vi "Open Hardware.vi"(8 "error in (no error)":errorcluster, 11 "Instrument.Oxford1820 in":refnum<class "Instrument.Oxford1820.lvclass">) -> (0 "error out":errorcluster, 3 "Instrument.Oxford1820 out":refnum<class "Instrument.Oxford1820.lvclass">)   [LabVIEW 2019, in "Instrument.Oxford1820.lvclass"]
uses:
  Instrument.Oxford1820.lvclass
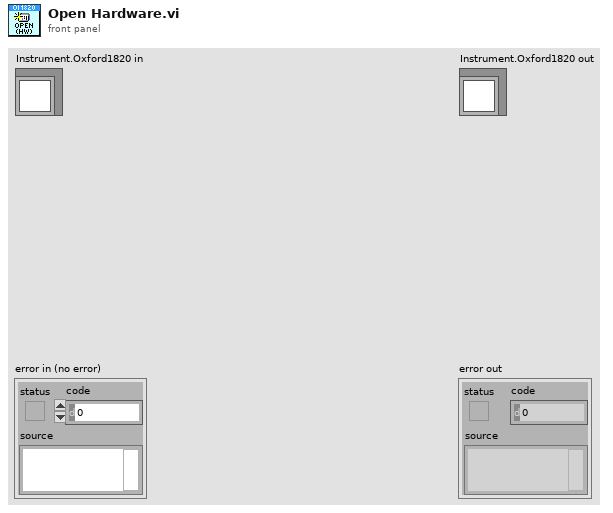
[diagram p1: front panel]
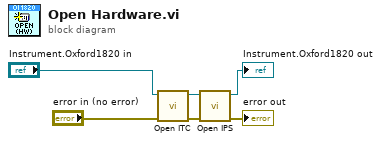
[diagram p0: block diagram]
diagram:
  n1 = call "Open ITC.vi"("error in (no error)"="error in (no error)", "Instrument.Oxford1820 in"="Instrument.Oxford1820 in") -> ("error out"=w2:errorcluster, "Instrument.Oxford1820 out"=w4:refnum<class "Instrument.Oxford1820.lvclass">)  [unwired: 8 in]
  n2 = call "Open IPS.vi"("error in (no error)"=w2, "Instrument.Oxford1820 in"=w4) -> ("error out"=→"error out":errorcluster, "Instrument.Oxford1820 out"=→"Instrument.Oxford1820 out":refnum<class "Instrument.Oxford1820.lvclass">)  [unwired: 8 in]
